vi "Finish.vi"(8 "error in (no error)":errorcluster, 11 "Simulated Drive in":refnum<class "Simulated Drive.lvclass">) -> (0 "error out":errorcluster, 3 "Simulated Drive out":refnum<class "Simulated Drive.lvclass">)   [LabVIEW 2019, in "DriveOld.lvlib" / "Simulated Drive.lvclass"]
doc: "Code that runs at the end"
uses:
  Simulated Drive.lvclass
  Drive.lvclass
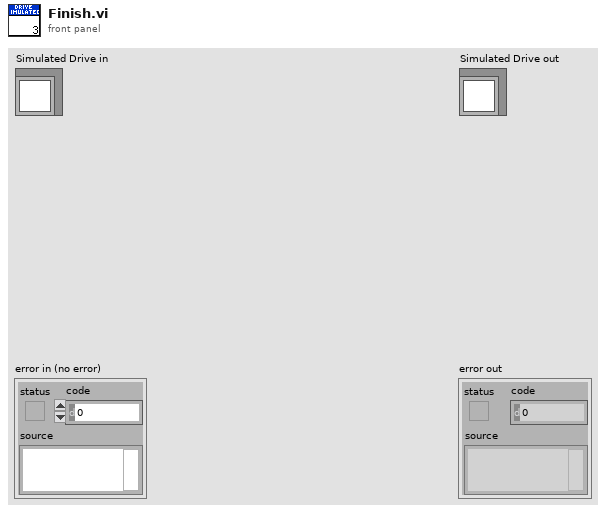
[diagram p1: front panel]
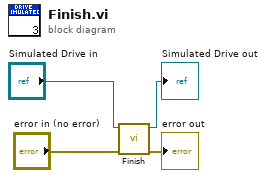
[diagram p0: block diagram]
diagram:
  n1 = call-parent "Finish.vi"("error in (no error)"="error in (no error)", "Drive in"="Simulated Drive in") -> ("error out"=→"error out":errorcluster, "Drive out"=→"Simulated Drive out":refnum<class "Simulated Drive.lvclass">)  [unwired: 8 in]
